vi "Init.vi"(8 "error in (no error)":errorcluster, 11 "UI Actor in":refnum<class "UI Actor.lvclass">) -> (0 "error out":errorcluster, 3 "UI Actor out":refnum<class "UI Actor.lvclass">)   [LabVIEW 2020, in "UI Actor.lvlib" / "UI Actor.lvclass"]
uses:
  UI Actor.lvclass
  C:/Program Files (x86)/National Instruments/LabVIEW 2020/vi.lib/ActorFramework/Actor/Actor.lvclass
  MSG/MSG.lvclass
  UI Actor.lvclass/UI Actor.ctl
  Soda Actor/Soda Actor.lvclass
  Soda Actor/Soda Actor.lvclass/Soda Actor.ctl
  Nestle Actor/Nestle Actor.lvclass
  Nestle Actor/Nestle Actor.lvclass/Nestle Actor.ctl
  MXN Actor/MXN Actor.lvclass
  MXN Actor/MXN Actor.lvclass/MXN Actor.ctl
  USD Actor/USD Actor.lvclass
  USD Actor/USD Actor.lvclass/USD Actor.ctl
  MSG/MSG.lvclass/MSG.ctl
  Read Coins.vi
  Read Sub Panel coin.vi
  Read Products.vi
  Read Sub Panel Prod.vi
  Read Sub Panel MSG.vi
  <vilib>/ActorFramework/Actor/Actor.lvclass
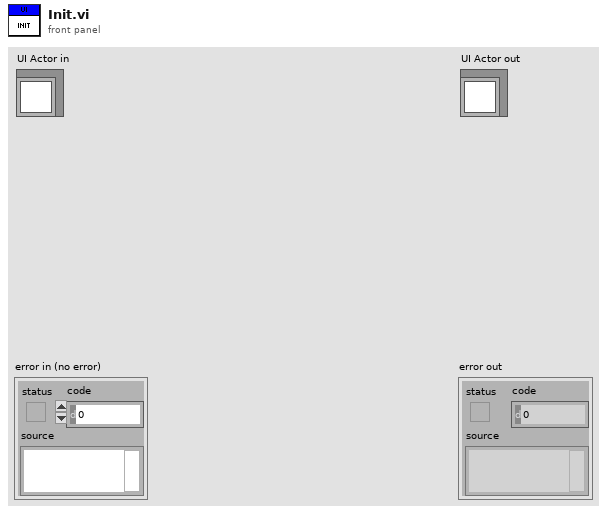
[diagram p1: front panel]
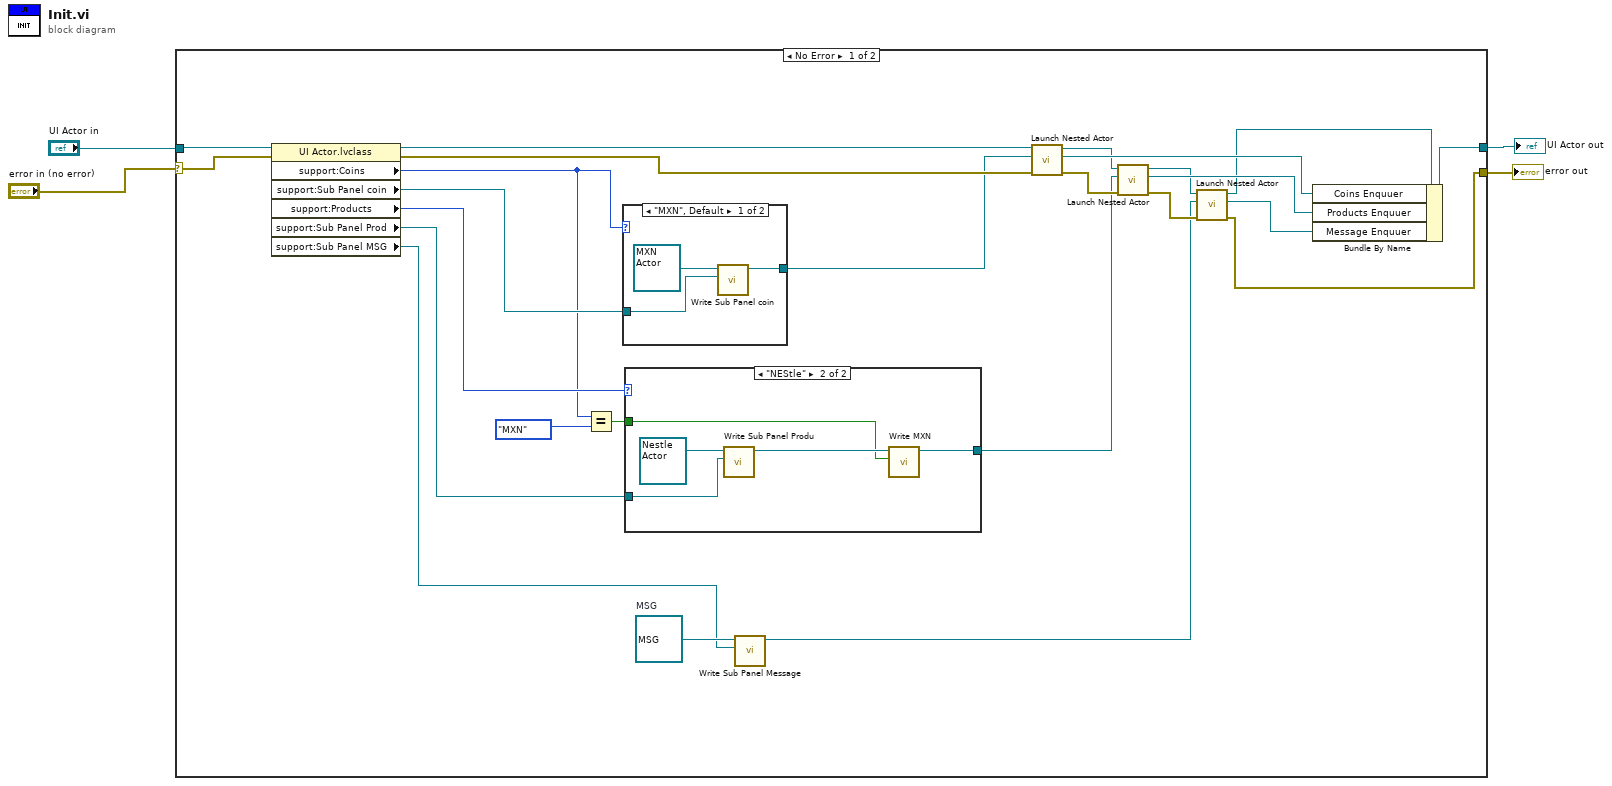
[diagram p0: block diagram]
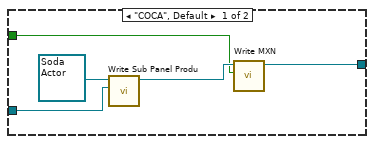
[diagram p2: hidden frame]
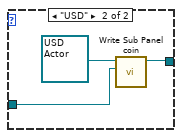
[diagram p3: hidden frame]
diagram:
  n1 = case shown="No Error" "error in (no error)" {
    selector: "error in (no error)" -> [w28 w47]
    tunnel: [w12 w47] -> w3
    tunnel: [w24 w46] -> w1
    tunnel: "UI Actor in" -> [w29 w46]
    frame No Error {
      w10 = refnum<class "MSG.lvclass"> refnum  # MSG
      n2 = property class="UI Actor.lvclass"(reference=w29, error in=w28) -> (reference out=w26:refnum<class "UI Actor.lvclass">, error out=w27:errorcluster, "support:Coins"=w7:enum16{"MXN", "USD"}, "support:Sub Panel coin"=w21:refnum<vi>, "support:Products"=w22:enum16{"COCA", "NEStle", ""}, "support:Sub Panel Prod"=w17:refnum<vi>, "support:Sub Panel MSG"=w9:refnum<vi>)
      n3 = Equal?(x=w7, y=enum16{"MXN", "USD"}."MXN" ("Coins")) -> (x = y?=w5:bool)
      n4 = case shown="\"MXN\", Default" w7 {
        tunnel: [w42 w45] -> w25
        tunnel: w21 -> [w40 w43]
        frame "MXN", Default {
          n5 = call "Write Sub Panel coin.vi"("Sub Panel coin"=w40, "MXN Actor in"=refnum<class "MXN Actor.lvclass"> refnum ("MXN Actor.lvlib:MXN Actor.lvclass")) -> ("MXN Actor out"=w42:refnum<class "MXN Actor.lvclass">)  [unwired: 8 in, 1 out]
        }
        frame "USD" {
          n6 = call "Write Sub Panel coin.vi"("Sub Panel coin"=w43, "USD Actor in"=refnum<class "USD Actor.lvclass"> refnum ("USD Actor.lvlib:USD Actor.lvclass")) -> ("USD Actor out"=w45:refnum<class "USD Actor.lvclass">)  [unwired: 8 in, 1 out]
        }
      }
      n7 = case shown="\"NEStle\"" w22 {
        tunnel: w17 -> [w33 w38]
        tunnel: [w31 w36] -> w18
        tunnel: w5 -> [w30 w35]
        frame "COCA", Default {
          n8 = call "Write Sub Panel Produ.vi"("Sub Panel Produ"=w33, "Soda Actor in"=refnum<class "Soda Actor.lvclass"> refnum ("Soda Actor.lvlib:Soda Actor.lvclass")) -> ("Soda Actor out"=w32:refnum<class "Soda Actor.lvclass">)  [unwired: 8 in, 1 out]
          n9 = call "Write MXN.vi"("MXN"=w30, "Soda Actor in"=w32) -> ("Soda Actor out"=w31:refnum<class "Soda Actor.lvclass">)  [unwired: 8 in, 1 out]
        }
        frame "NEStle" {
          n10 = call "Write Sub Panel Produ.vi"("Sub Panel Produ"=w38, "Nestle Actor in"=refnum<class "Nestle Actor.lvclass"> refnum ("Nestle Actor.lvlib:Nestle Actor.lvclass")) -> ("Nestle Actor out"=w37:refnum<class "Nestle Actor.lvclass">)  [unwired: 8 in, 1 out]
          n11 = call "Write MXN.vi"("MXN"=w35, "Nestle Actor in"=w37) -> ("Nestle Actor out"=w36:refnum<class "Nestle Actor.lvclass">)  [unwired: 8 in, 1 out]
        }
      }
      n12 = call "Write Sub Panel Message.vi"("Sub Panel Message"=w9, "MSG in"=w10) -> ("MSG out"=w8:refnum<class "MSG.lvclass">)  [unwired: 8 in, 1 out]
      n13 = call <vilib>:"Launch Nested Actor.vi"("error in (no error)"=w27, "Nested Actor"=w25, "Caller Actor in"=w26) -> ("error out"=w19:errorcluster, "Nested Actor's Enqueuer"=w23:refnum<class "Message Enqueuer.lvclass">, "Caller Actor out"=w20:refnum<class "UI Actor.lvclass">)  [unwired: 6 in]
      n14 = call <vilib>:"Launch Nested Actor.vi"("error in (no error)"=w19, "Nested Actor"=w18, "Caller Actor in"=w20) -> ("error out"=w13:errorcluster, "Nested Actor's Enqueuer"=w16:refnum<class "Message Enqueuer.lvclass">, "Caller Actor out"=w15:refnum<class "UI Actor.lvclass">)  [unwired: 6 in]
      n15 = call <vilib>:"Launch Nested Actor.vi"("error in (no error)"=w13, "Nested Actor"=w8, "Caller Actor in"=w15) -> ("error out"=w12:errorcluster, "Nested Actor's Enqueuer"=w11:refnum<class "Message Enqueuer.lvclass">, "Caller Actor out"=w14:refnum<class "UI Actor.lvclass">)  [unwired: 6 in]
      n16 = Bundle By Name(cluster=w14, "Coins Enquuer"=w23, "Products Enquuer"=w16, "Message Enquuer"=w11) -> (w24:refnum<class "UI Actor.lvclass">)
    }
    frame Error {
    }
  }
  "error out" <- w3
  "UI Actor out" <- w1
